vi "FGV Leitstand.vi"(6 "Aktionen":T1, 10 "Kühlung FT-IR aktiv/inaktiv":u16) -> (2 "Kühlung FT-IR aktiv/inaktiv":u16)   [LabVIEW 2020, in "Erweiterte Konfig.lvlib"]
uses:
  Erweiterte Konfig.lvlib
  Aktioen FGV Leitstand.ctl
  Allgemein/allgemeine Sub-VIs.lvlib
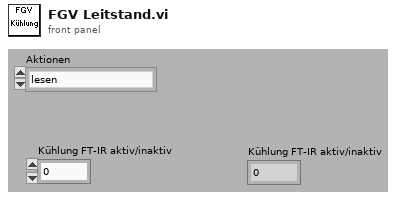
[diagram p1: front panel]
types:
  T1 = typedef "Erweiterte Konfig.lvlib/Aktioen FGV Leitstand.ctl" = enum16{"lesen", "laden", "speichern", "schreiben"}
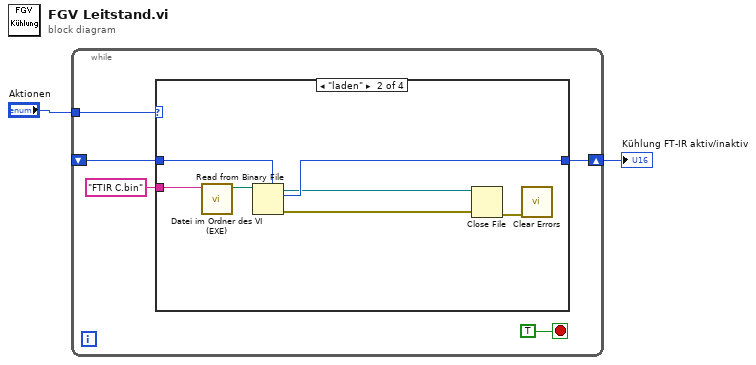
[diagram p0: block diagram]
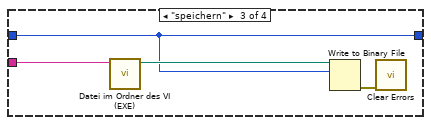
[diagram p3: hidden frame]
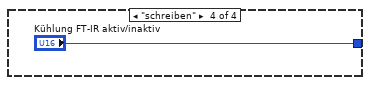
[diagram p4: hidden frame]
diagram:
  n1 = while {
    shift-right: [w4] -> w1
    shift-left: _ -> [w5]
    tunnel: "Aktionen" -> [w6]
    stop <- TRUE stop-if-true
    n2 = case shown="\"laden\"" w6 {
      tunnel: w5 -> [w8 w14 w18 _]
      tunnel: [w8 w13 w18 "Kühlung FT-IR aktiv/inaktiv"] -> w4
      tunnel: "FTIR C.bin" ("Dateiname") -> [_ w12 w16 _]
      frame "lesen", Default {
      }
      frame "laden" {
        n3 = call "Datei im Ordner des VI (EXE).vi"("Dateiname"=w12) -> ("Dateipfad im Ordner des Haupt-VIs"=w15:path)  [unwired: 8 in, 2 out]
        n4 = Read from Binary File(5:w14, 11:w15) -> (0:w11:errorcluster, 2:w13:u16, 3:w9:refnum<file>)  [unwired: 1 in, 4 out]
        n5 = Close File(refnum=w9, error in=w11) -> (error out=w10:errorcluster)  [unwired: 1 out]
        n6 = call <vilib>:"Clear Errors.vi"("error in (no error)"=w10) -> ()  [unwired: 5 in, 2 out]
      }
      frame "speichern" {
        n7 = call "Datei im Ordner des VI (EXE).vi"("Dateiname"=w16) -> ("Dateipfad im Ordner des Haupt-VIs"=w19:path)  [unwired: 8 in, 2 out]
        n8 = Write to Binary File(file (use dialog)=w19, data=w18) -> (error out=w17:errorcluster)  [unwired: 1 in, 5 out]
        n9 = call <vilib>:"Clear Errors.vi"("error in (no error)"=w17) -> ()  [unwired: 5 in, 2 out]
      }
      frame "schreiben" {
      }
    }
  }
  "Kühlung FT-IR aktiv/inaktiv" <- w1
